vi "OBJECT DETECTOR AND ENCRYPTOR.vi"() -> ()   [LabVIEW 2023]
uses:
  <vilib>/vision/Deep Learning.llb/IMAQ DL Model Type.ctl
  <vilib>/userDefined/High Color/IMAQdx.ctl
  <vilib>/vision/Deep Learning.llb/IMAQ DL Model Detect Objects Node Names.ctl
  <vilib>/vision/Deep Learning.llb/IMAQ DL Model Label.ctl
  <vilib>/vision/NI_Vision_Development_Module.lvlib
  <vilib>/vision/driver/NI_Vision_Acquisition_Software.lvlib
panel:
  in  "OBJETOS A ENCRIPTAR":string(combo)
  in  "stop":bool
  out "Inspection Image":T1(plugin-control)
  out "Image":T1(plugin-control)
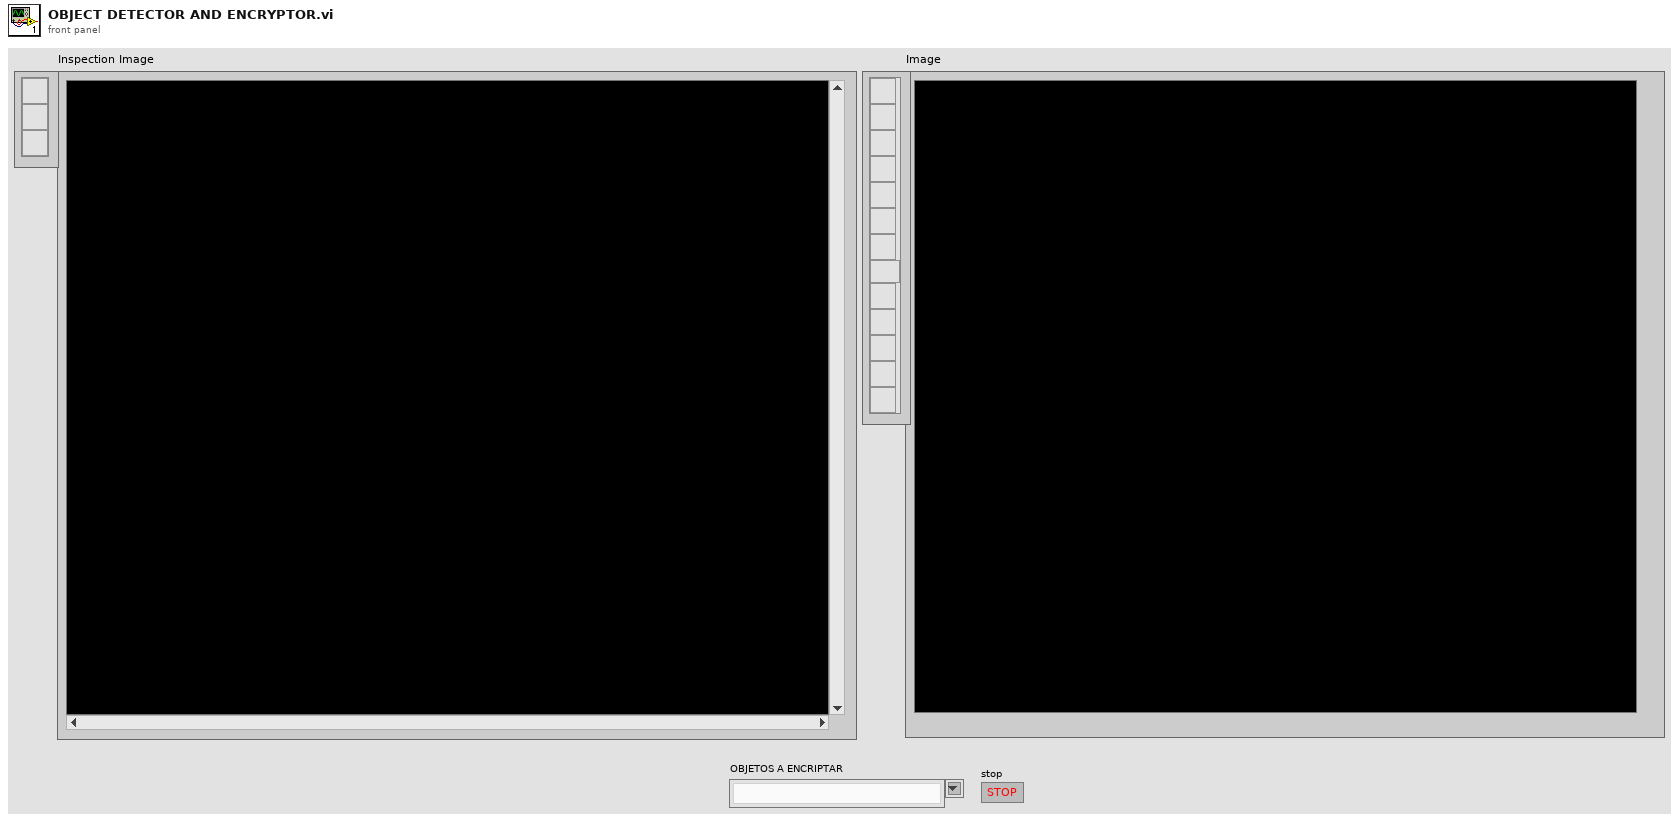
[diagram p1: front panel]
types:
  T1 = typedef "IMAQ Image.ctl" = refnum<image>
  T2 = typedef "Image Type" = u32
  T3 = typedef "IMAQdx.ctl" = refnum<k21>
  T4 = typedef "IMAQ DL Model Type.ctl" = i32
  T5 = typedef "IMAQ DL Model Refnum.ctl" = refnum<k20>
  T6 = typedef "IMAQ DL Model Label.ctl" = cluster{"ID":u32, "Label":string}
  T7 = typedef "IMAQ DL Model Detect Objects Node Names.ctl" = cluster{"Number of Objects":string, "Labels":string, "Scores":string, "Bounding Boxes":string}
  T8 = typedef "IMAQ DL Model Objects.ctl" = cluster{"Label":string, "Score":sgl, "Bounding Box":cluster{"x":sgl, "y":sgl}[]}
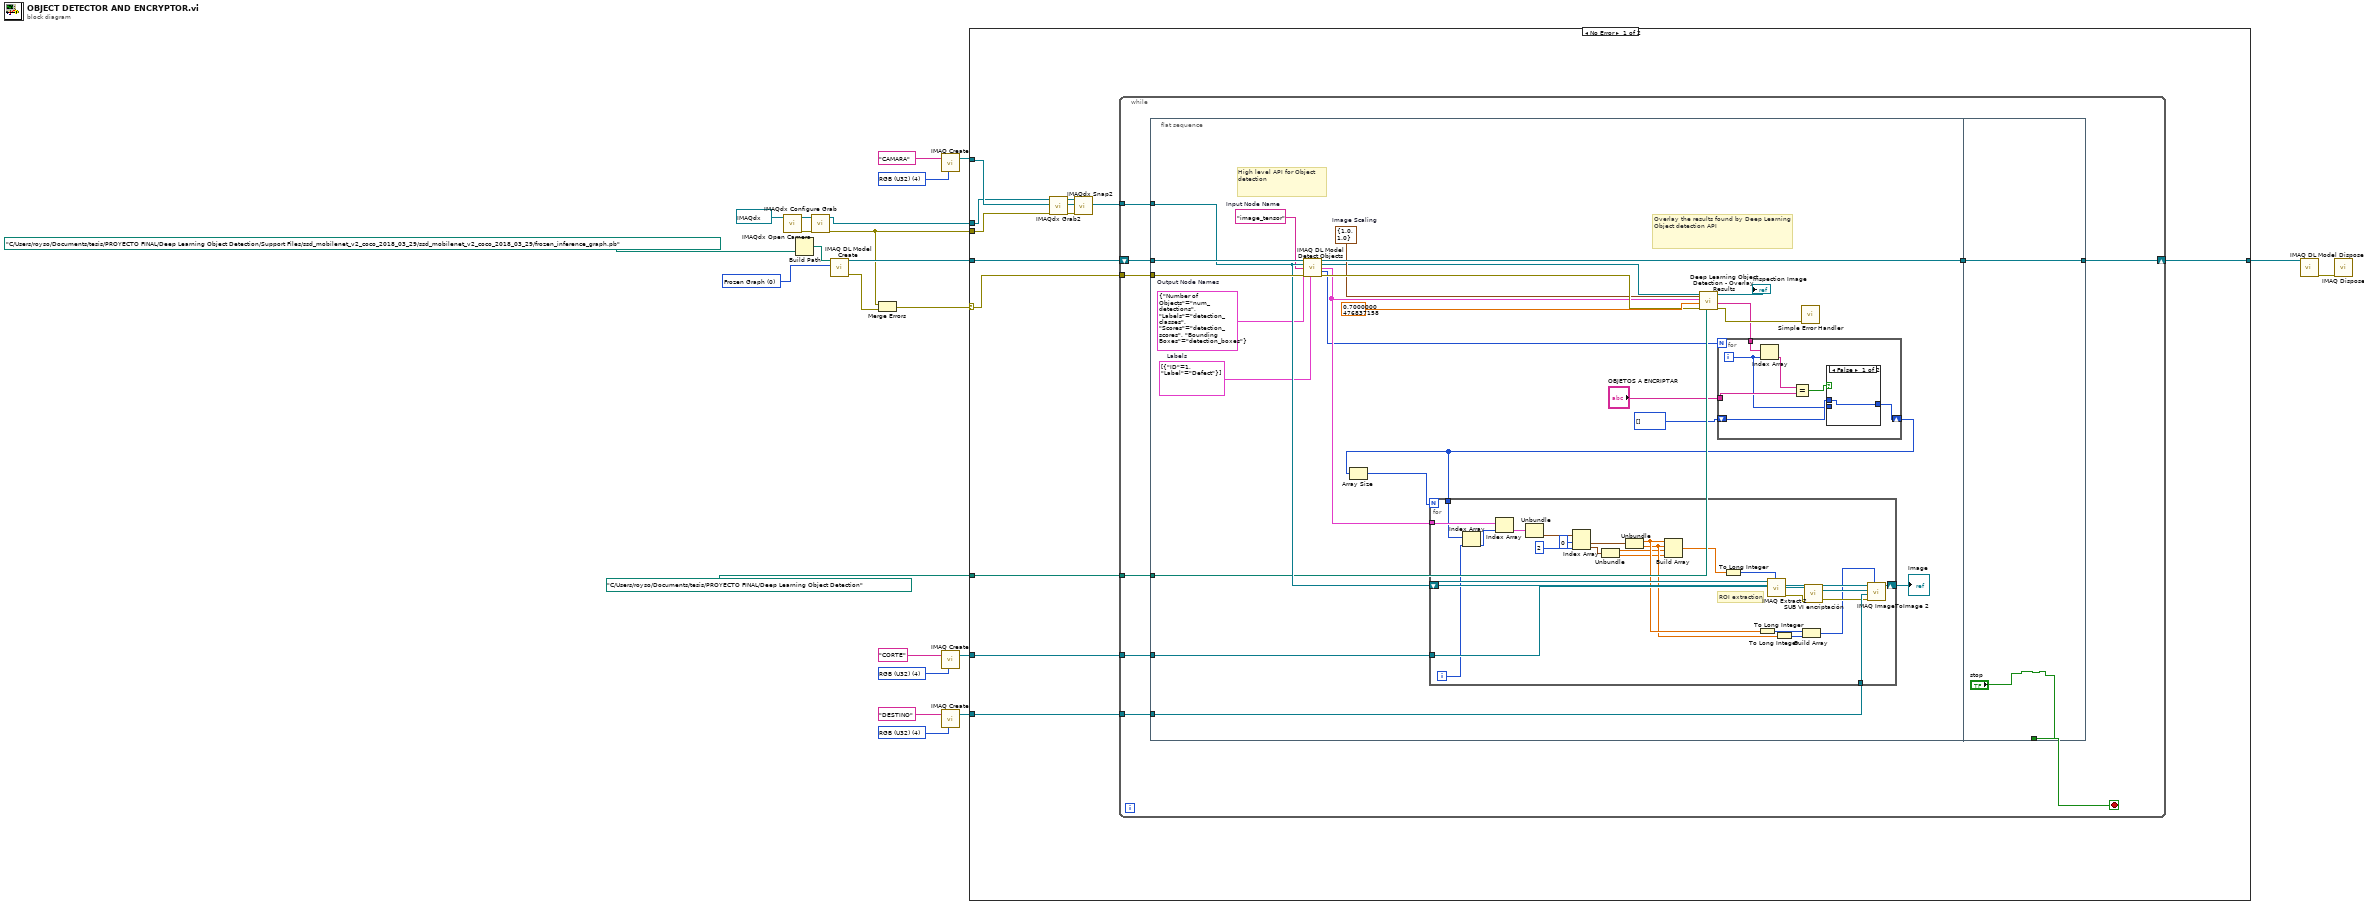
[diagram p0: block diagram]
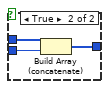
[diagram p2: hidden frame]
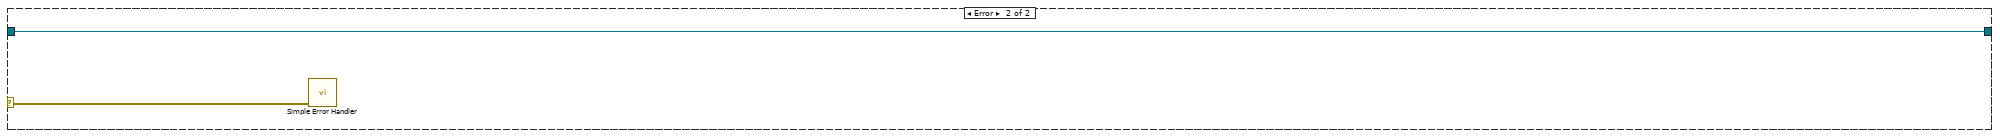
[diagram p3: hidden frame]
diagram:
  w2 = T2 4 items=["Grayscale (U8)", "Grayscale (I16)", "Grayscale (SGL)", "Complex (CSG)", "RGB (U32)", "HSL (U32)", "RGB (U64)", "Grayscale (U16)"] ("Image Type")
  w13 = T2 4 items=["Grayscale (U8)", "Grayscale (I16)", "Grayscale (SGL)", "Complex (CSG)", "RGB (U32)", "HSL (U32)", "RGB (U64)", "Grayscale (U16)"] ("Image Type")
  w15 = T2 4 items=["Grayscale (U8)", "Grayscale (I16)", "Grayscale (SGL)", "Complex (CSG)", "RGB (U32)", "HSL (U32)", "RGB (U64)", "Grayscale (U16)"] ("Image Type")
  w19 = T4 0 items=["Frozen Graph", "Saved Model"] ("Model Type")
  n1 = call <vilib>:"IMAQdx Open Camera.vi"("Session In"=T3 "cam2") -> ("error out"=w8:errorcluster, "Session Out"=w9:T3)  [unwired: 9 in]
  n2 = Build Path(name or relative path=path "C:/Users/royso/Documents/tesis/PROYECTO FINAL/Deep Learning Object Detection/Support Files/ssd_mobilenet_v2_coco_2018_03_29/ssd_mobilenet_v2_coco_2018_03_29/frozen_inference_graph.pb") -> (appended path=w23:path)  [unwired: 1 in]
  n3 = call <vilib>:"IMAQdx Configure Grab.vi"("error in"=w8, "Session In"=w9) -> ("error out"=w4:errorcluster, "Session Out"=w5:T3)  [unwired: 8 in]
  n4 = call-poly "IMAQ DL Model Create"("Model Type"=w19, "File Path"=w23) -> ("error out"=w20:errorcluster, "Model Refnum"=w22:T5)  [unwired: 8 in]
  n5 = Merge Errors(w4, w20) -> (w3:errorcluster)
  n6 = call "IMAQ Create"("Image Name"="CAMARA", "Image Type"=w2) -> ("New Image"=w6:T1)  [unwired: 3 in, 1 out]
  n7 = call "IMAQ Create"("Image Name"="CORTE", "Image Type"=w15) -> ("New Image"=w12:T1)  [unwired: 3 in, 1 out]
  n8 = call "IMAQ Create"("Image Name"="DESTINO", "Image Type"=w13) -> ("New Image"=w11:T1)  [unwired: 3 in, 1 out]
  n9 = case shown="No Error" w3 {
    selector: w3 -> [w34 w110]
    tunnel: w22 -> [w36 w111]
    tunnel: [w35 w111] -> w21
    tunnel: w12 -> [w33 _]
    tunnel: w11 -> [w32 _]
    tunnel: w6 -> [w29 _]
    tunnel: w5 -> [w28 _]
    tunnel: w4 -> [w30 _]
    tunnel: path "C:/Users/royso/Documents/tesis/PROYECTO FINAL/Deep Learning Object Detection" ("base path") -> [w31 _]
    frame No Error {
      n10 = call <vilib>:"IMAQdx Grab2.vi"("error in"=w30, "Image In"=w29, "Session In"=w28) -> ("error out"=w26:errorcluster, "Image Out"=w25:T1, "Session Out"=w24:T3)  [unwired: 5 in, 1 out]
      n11 = call <vilib>:"IMAQdx Snap2.vi"("error in"=w26, "Image In"=w25, "Session In"=w24) -> ("Image Out"=w27:T1)  [unwired: 6 in, 2 out]
      n12 = while {
        tunnel: w34 -> [w43]
        tunnel: w33 -> [w42]
        tunnel: w32 -> [w41]
        tunnel: w27 -> [w40]
        tunnel: w31 -> [w39]
        shift-right: [w44] -> w35
        shift-left: w36 -> [w45]
        stop <- w37 stop-if-true
        n13 = flat-sequence {
          tunnel: w45 -> [w69]
          tunnel: w43 -> [w67]
          tunnel: w42 -> [w66]
          tunnel: w41 -> [w65]
          tunnel: w40 -> [w64]
          tunnel: w39 -> [w63]
          tunnel: [w68] -> w38
          tunnel: [w109] -> w44
          tunnel: w38 -> [w109]
          tunnel: ["stop"] -> w37
          frame #0 {
            w56 = T6[] [{"ID"=1, "Label"="Defect"}]  # Labels
            w58 = T7 {"Number of Objects"="num_detections", "Labels"="detection_classes", "Scores"="detection_scores", "Bounding Boxes"="detection_boxes"}  # Output Node Names
            w59 = "image_tensor"  # Input Node Name
            w60 = cluster{"X":dbl, "Y":dbl} {"X"=1.0, "Y"=1.0}  # Image Scaling
            # "Overlay the results found by Deep Learning  Object detection API"
            # "High level API for Object detection"
            n14 = call "IMAQ DL Model Detect Objects"("Model Refnum In"=w69, "Image"=w64, "Input Node Name"=w59, "Output Node Names"=w58, "error in (no error)"=w67, "Labels"=w56) -> ("Model Refnum Out"=w68:T5, "Image (duplicate)"=w53:T1, "Detected Objects"=w55:T8[], "Number of Objects"=w51:i32, "error out"=w61:errorcluster)  [unwired: 5 in]
            n15 = call "Deep Learning Object Detection - Overlay Results.vi"("base path"=w63, "Image Scaling"=w60, "error in (no error)"=w61, "Minimum Score Threshold"=sgl 0.70000005, "Detected Objects"=w55, "Image In"=w53) -> ("error out"=w57:errorcluster, "Array"=w50:string[], "Image Out"=→"Inspection Image":T1)  [unwired: 3 in]
            n16 = for {
              N: w51 -> [_]
              tunnel: w50 -> [w103]
              tunnel: "OBJETOS A ENCRIPTAR" -> [w101]
              shift-right: [w97] -> w46
              shift-left: i32[] [] -> [w99]
              i -> [w98]
              n17 = Index Array(array=w103, index=w98) -> (element=w102:string)
              n18 = Equal?(x=w102, y=w101) -> (x = y?=w100:bool)
              n19 = case shown="False" w100 {
                tunnel: w99 -> [w104 w107]
                tunnel: w98 -> [_ w106]
                tunnel: [w104 w105] -> w97
                frame False {
                }
                frame True {
                  n20 = Build Array (concatenate)(w107, w106) -> (w105:i32[])
                }
              }
            }
            n21 = Array Size(array=w46) -> (size(s)=w48:i32)
            n22 = for {
              N: w48 -> [_]
              tunnel: w66 -> [w96]
              tunnel: w65 -> [w95]
              tunnel: w55 -> [w89]
              shift-right: [w73] -> w52
              shift-left: w64 -> [w94]
              tunnel: w46 -> [w71]
              i -> [w72]
              # "ROI extraction"
              n23 = Index Array(array=w71, index=w72) -> (element=w70:i32)
              n24 = Index Array(array=w89, index=w70) -> (element=w90:T8)
              n25 = Unbundle(w90) -> ("Bounding Box"=w93:cluster{"x":sgl, "y":sgl}[])  [unwired: 2 out]
              n26 = Index Array(array=w93, index #1=0 ("index"), index #2=2 ("index")) -> (element #1=w81:cluster{"x":sgl, "y":sgl}, element #2=w82:cluster{"x":sgl, "y":sgl})
              n27 = Unbundle(w82) -> ("x"=w77:sgl, "y"=w78:sgl)
              n28 = Unbundle(w81) -> ("x"=w80:sgl, "y"=w79:sgl)
              n29 = Build Array(w80, w79, w77, w78) -> (w88:sgl[])
              n30 = To Long Integer(number=w88) -> (32bit integer=w87:i32[])
              n31 = To Long Integer(number=w80) -> (32bit integer=w76:i32)
              n32 = call "IMAQ Extract 2"("Optional Rectangle"=w87, "Image Dst"=w96, "Image Src"=w94) -> ("error out"=w85:errorcluster, "Image Dst Out"=w86:T1)  [unwired: 7 in]
              n33 = To Long Integer(number=w79) -> (32bit integer=w75:i32)
              n34 = Build Array(w76, w75) -> (w74:i32[])
              n35 = call "SUB VI encriptación.vi"("error in (no error)"=w85, "Image 2"=w86) -> ("error out"=w83:errorcluster, "Image"=w84:T1)  [unwired: 7 in, 1 out]
              n36 = call "IMAQ ImageToImage 2"("Offset Left/Top"=w74, "error in (no error)"=w83, "Image Dst"=w95, "Image Src (Small)"=w84, "Image Src (Large)"=w94) -> ("Image Dst Out"=w73:T1)  [unwired: 5 in, 1 out]
            }
            "Image" <- w52
            n37 = call <vilib>:"Simple Error Handler.vi"("error in (no error)"=w57) -> ()  [unwired: 4 in, 5 out]
          }
          frame #1 {
          }
        }
      }
    }
    frame Error {
      n38 = call <vilib>:"Simple Error Handler.vi"("error in (no error)"=w110) -> ()  [unwired: 4 in, 5 out]
    }
  }
  n39 = call "IMAQ DL Model Dispose"("Model Refnum"=w21) -> ("error out"=w18:errorcluster)  [unwired: 10 in]
  n40 = call "IMAQ Dispose"("error in (no error)"=w18) -> ()  [unwired: 5 in, 1 out]
